vi "Do-Fft-Fpga-Top-Level.vi"() -> ()   [LabVIEW 2014]
uses:
  <vilib>/FPGA/interface/niFpgaViExecutionMode.ctl
panel:
  out "FPGA VI Execution Mode":T1
  out "Comparison failed at\nindex:":i32
  out "Results Match!":bool
  out "Results Filename":string
  out "Expected Results (truncated)":csg[](array[numeric])
  out "size(s)":i32
  in  "SourceFileName":string="data_16_1.txt"
  out "Results":csg[](array[numeric])
  out "error out":errorcluster
  out "Complex Data (in)":csg[](array[numeric])
  in  "error in":errorcluster
  # "<===== 1 value does not match"
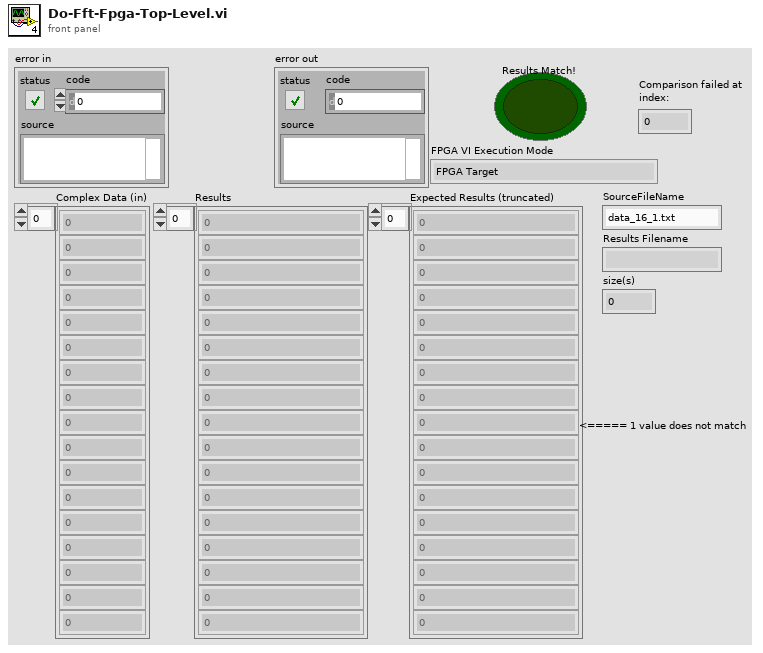
[diagram p1: front panel]
types:
  T1 = typedef "niFpgaViExecutionMode.ctl" = enum16{"FPGA Target", "Simulation (Simulated I/O)", "Simulation (Real I/O)", "Third-Party Simulation"}
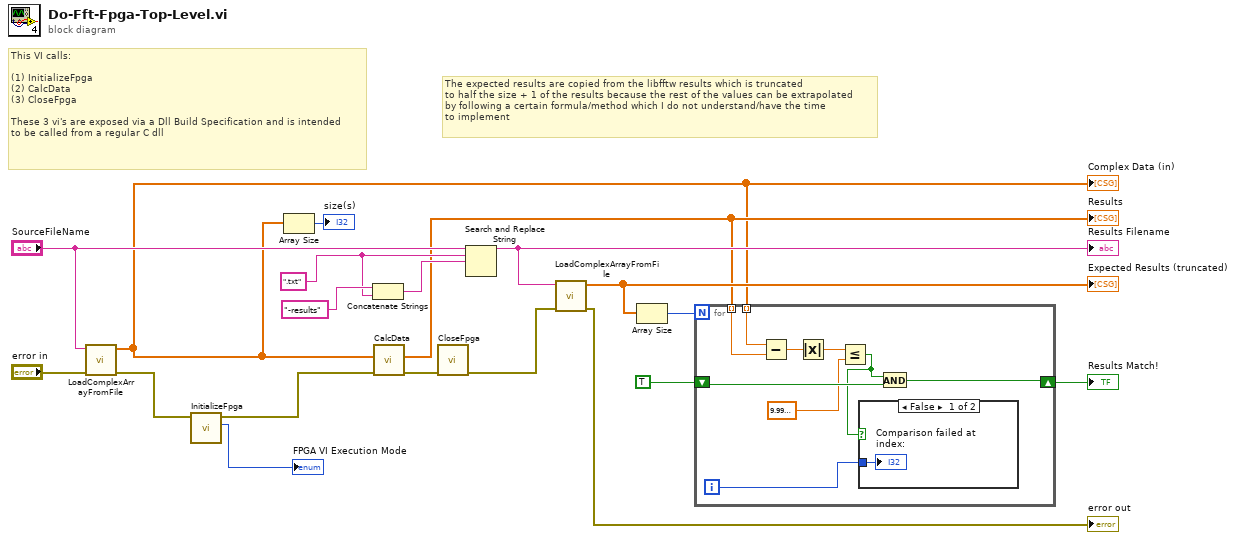
[diagram p0: block diagram]
diagram:
  w8 = ".txt" ("substring (\"\")")
  # "The expected results are copied from the libfftw results which is truncated\nto half the size + 1 of the results because the rest of the values can be extrapolated\nby following a certain formula/method which I do not understand/have the time\nto implement"
  # "This VI calls:\n\n(1) InitializeFpga\n(2) CalcData\n(3) CloseFpga\n\nThese 3 vi's are exposed via a Dll Build Specification and is intended\nto be called from a regular C dll"
  n1 = call "LoadComplexArrayFromFile.vi"("error in"="error in", "SourceFileName"="SourceFileName") -> ("error out"=w16:errorcluster, "Array"=w2:csg[])  [unwired: 8 in]
  "Complex Data (in)" <- w2
  n2 = call "InitializeFpga.vi"("error in"=w16) -> ("FPGA VI Execution Mode"=→"FPGA VI Execution Mode":T1, "error out"=w19:errorcluster)  [unwired: 9 in]
  n3 = Array Size(array=w2) -> (size(s)=→"size(s)":i32)
  n4 = Concatenate Strings("-results" ("replace string (\"\")"), w8) -> (w10:string)
  n5 = call "CalcData.vi"("error in (no error)"=w19, "Complex Data (in)"=w2) -> ("error out"=w18:errorcluster, "Array out"=w3:csg[])  [unwired: 8 in]
  "Results" <- w3
  n6 = call "CloseFpga.vi"("error in"=w18) -> ("error out"=w12:errorcluster)  [unwired: 10 in]
  n7 = Search and Replace String(input string="SourceFileName", search string=w8, replace string=w10) -> (result string=w13:string)  [unwired: 5 in, 3 out]
  "Results Filename" <- w13
  n8 = call "LoadComplexArrayFromFile.vi"("error in"=w12, "SourceFileName"=w13) -> ("error out"=→"error out":errorcluster, "Array"=w7:csg[])  [unwired: 8 in]
  "Expected Results (truncated)" <- w7
  n9 = Array Size(array=w7) -> (size(s)=w6:i32)
  n10 = for {
    N: w6 -> [_]
    shift-right: [w28] -> w4
    shift-left: TRUE -> [w27]
    tunnel: w3 -> [w25] mode=indexing
    tunnel: w2 -> [w26] mode=indexing
    i -> [w20]
    n11 = Subtract(x=w26, y=w25) -> (x-y=w24:csg)
    n12 = Absolute Value(x=w24) -> (abs(x)=w23:sgl)
    n13 = Less Or Equal?(x=w23, y=sgl 1e-08) -> (x <= y?=w21:bool)
    n14 = case shown="False" w21 {
      tunnel: w20 -> [w29 _]
      frame False {
        "Comparison failed at\nindex:" <- w29
      }
      frame True {
      }
    }
    n15 = And(x=w21, y=w27) -> (x .and. y?=w28:bool)
  }
  "Results Match!" <- w4
